vi "Detect Conflicts.vi"(8 "error in (no error)":errorcluster, 10 "roboRIO":path, 11 "Local":path) -> (0 "error out":errorcluster, 1 "Conflicts?":bool, 2 "roboRIO out":path, 3 "Local out":path, 5 "Items with conflicts":T1[](array[typedef]))   [LabVIEW 2018, in "Personalities Tool.lvlib"]
doc: "This VI reads both configuration files and detects conflicts with missing keys, or different information."
uses:
  Personalities Tool.lvlib
  Controls/Diff Key.ctl
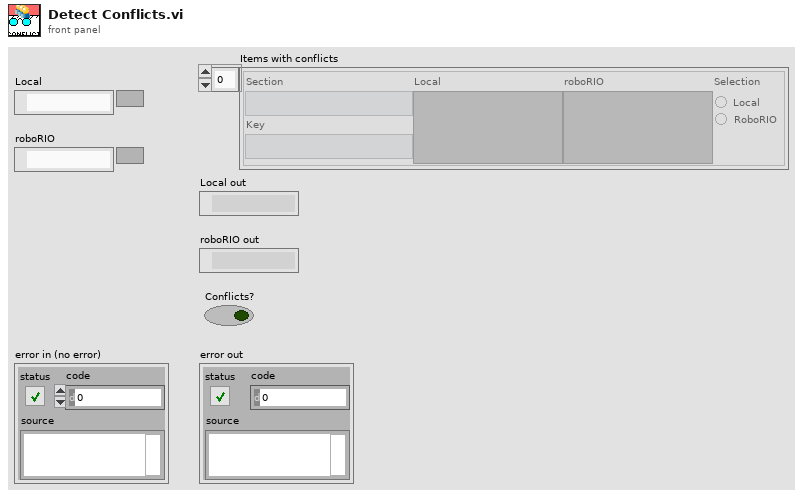
[diagram p1: front panel]
types:
  T1 = typedef "Personalities Tool.lvlib/Diff Key.ctl" = cluster{"Section":string, "Local":variant, "roboRIO":variant, "Selection":enum32{"Item 0", "Item 1"}, "Key":string}
  T2 = typedef "Personalities Tool.lvlib/Sections and keys.ctl" = cluster{"Section names":string[], "Keys and values per section":variant[]}
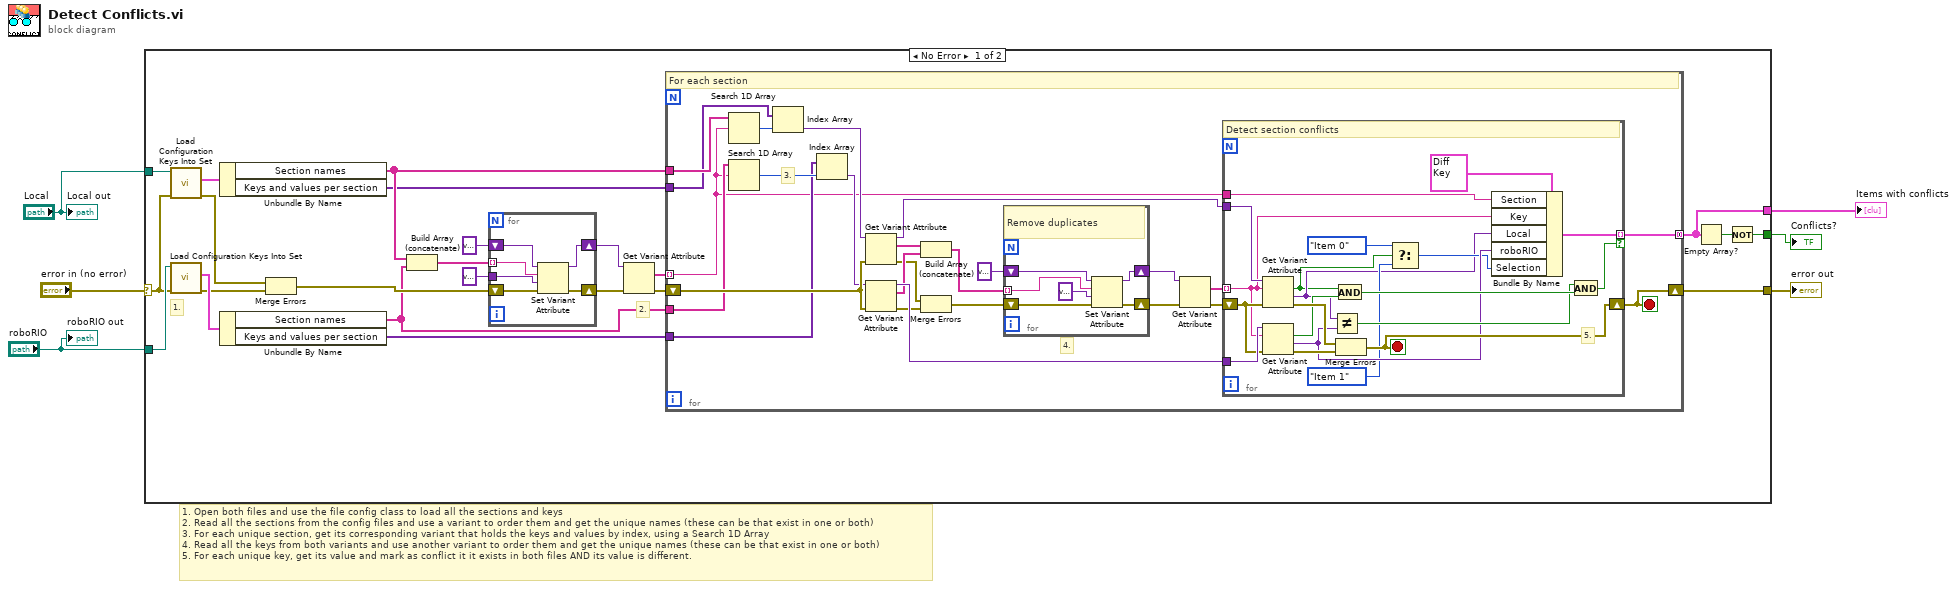
[diagram p0: block diagram]
diagram:
  # "1. Open both files and use the file config class to load all the sections and keys\n2. Read all the sections from the config files and use a variant to order them and get the unique names (these can be that exist in one or both)\n3. For each unique section, get its corresponding variant that holds the keys and values by index, using a Search 1D Array\n4. Read all the keys from both variants and use another variant to order them and get the unique names (these can be that exist in one or both)\n5. For each unique key, get its value and mark as conflict it it exists in both files AND its value is different."
  n1 = case shown="No Error" "error in (no error)" {
    selector: "error in (no error)" -> [w24 w87]
    tunnel: [w29 _] -> w6
    tunnel: [w27 _] -> w5
    tunnel: [w26 w87] -> w4
    tunnel: "roboRIO" -> [w25 _]
    tunnel: "Local" -> [w23 _]
    frame No Error {
      # "2."
      # "1."
      n2 = call "Load Configuration Keys Into Set.vi"("error in (no error)"=w24, "Path"=w23) -> ("error out"=w18:errorcluster, "Sections and keys"=w21:T2)  [unwired: 7 in, 1 out]
      n3 = call "Load Configuration Keys Into Set.vi"("error in (no error)"=w24, "Path"=w25) -> ("error out"=w17:errorcluster, "Sections and keys"=w20:T2)  [unwired: 7 in, 1 out]
      n4 = Unbundle By Name(w21) -> ("Section names"=w11:string[], "Keys and values per section"=w8:variant[])
      n5 = Unbundle By Name(w20) -> ("Section names"=w10:string[], "Keys and values per section"=w9:variant[])
      n6 = Merge Errors(w18, w17) -> (w16:errorcluster)
      n7 = Build Array (concatenate)(w11, w10) -> (w19:string[])
      n8 = for {
        tunnel: w19 -> [w34] mode=indexing
        shift-right: [w33] -> w15
        shift-left: variant ("variant") -> [w35]
        shift-right: [w31] -> w14
        shift-left: w16 -> [w32]
        tunnel: variant -> [w30]
        n9 = Set Variant Attribute(Variant=w35, name=w34, value=w30, error in=w32) -> (Variant out=w33:variant, error out=w31:errorcluster)  [unwired: 1 out]
      }
      n10 = Get Variant Attribute(Variant=w15, error in=w14) -> (names=w12:string[], error out=w13:errorcluster)  [unwired: 2 in, 2 out]
      n11 = for {
        tunnel: [w60] -> w27 mode=concatenating
        shift-right: [w37] -> w26
        shift-left: w13 -> [w46]
        tunnel: w12 -> [w36] mode=indexing
        tunnel: w11 -> [w45]
        tunnel: w10 -> [w44]
        tunnel: w9 -> [w41]
        tunnel: w8 -> [w40]
        stop <- w37 stop-if-true
        # "4."
        # "3."
        # "For each section"
        n12 = Search 1D Array(1D array=w45, element=w36) -> (index of element=w43:i32)  [unwired: 1 in]
        n13 = Search 1D Array(1D array=w44, element=w36) -> (index of element=w42:i32)  [unwired: 1 in]
        n14 = Index Array(array=w40, index=w43) -> (element=w39:variant)
        n15 = Index Array(array=w41, index=w42) -> (element=w38:variant)
        n16 = Get Variant Attribute(Variant=w39, error in=w46) -> (duplicate Variant=w52:variant, names=w50:string[], error out=w49:errorcluster)  [unwired: 2 in, 1 out]
        n17 = Get Variant Attribute(Variant=w38, error in=w46) -> (duplicate Variant=w53:variant, names=w51:string[], error out=w48:errorcluster)  [unwired: 2 in, 1 out]
        n18 = Build Array (concatenate)(w50, w51) -> (w55:string[])
        n19 = Merge Errors(w49, w48) -> (w54:errorcluster)
        n20 = for {
          tunnel: w55 -> [w66] mode=indexing
          shift-right: [w63] -> w57
          shift-left: variant ("variant") -> [w62]
          shift-right: [w64] -> w56
          shift-left: w54 -> [w65]
          # "Remove duplicates"
          n21 = Set Variant Attribute(Variant=w62, name=w66, value=variant ("variant"), error in=w65) -> (Variant out=w63:variant, error out=w64:errorcluster)  [unwired: 1 out]
        }
        n22 = Get Variant Attribute(Variant=w57, error in=w56) -> (names=w58:string[], error out=w47:errorcluster)  [unwired: 2 in, 2 out]
        n23 = for {
          tunnel: w58 -> [w78] mode=indexing
          shift-right: [w83] -> w37
          shift-left: w47 -> [w84]
          tunnel: [w79] -> w60 mode=indexing if=w75
          tunnel: w52 -> [w86]
          tunnel: w53 -> [w85]
          tunnel: w36 -> [w67]
          stop <- w83 stop-if-true
          # "5."
          # "Detect section conflicts"
          n24 = Get Variant Attribute(Variant=w86, name=w78, error in=w84) -> (found=w68:bool, value=w69:variant, error out=w81:errorcluster)  [unwired: 1 in, 1 out]
          n25 = Get Variant Attribute(Variant=w85, name=w78, error in=w84) -> (found=w77:bool, value=w73:variant, error out=w82:errorcluster)  [unwired: 1 in, 1 out]
          n26 = Not Equal?(x=w69, y=w73) -> (x != y?=w74:bool)
          n27 = And(x=w68, y=w77) -> (x .and. y?=w76:bool)
          n28 = Merge Errors(w81, w82) -> (w83:errorcluster)
          n29 = Select(t=enum32{"Item 0", "Item 1"}."Item 0" ("Selection"), s=w68, f=enum32{"Item 0", "Item 1"}."Item 1" ("Selection")) -> (s? t:f=w71:enum32{"Item 0", "Item 1"})
          n30 = Bundle By Name(cluster=T1 {"Section"="", "Local"=variant(string ""), "roboRIO"=variant(string ""), "Selection"=enum."Item 0", "Key"=""} ("Key Diff"), "Section"=w67, "Key"=w78, "Local"=w69, "roboRIO"=w73, "Selection"=w71) -> (w79:T1)
          n31 = And(x=w74, y=w76) -> (x .and. y?=w75:bool)
        }
      }
      n32 = Empty Array?(array=w27) -> (empty?=w28:bool)
      n33 = Not(x=w28) -> (.not. x?=w29:bool)
    }
    frame Error {
    }
  }
  "Conflicts?" <- w6
  "Items with conflicts" <- w5
  "error out" <- w4
  "roboRIO out" <- "roboRIO"
  "Local out" <- "Local"
